vi "通用文件传.vi"(5 "原文件路径（使用对话框）":path) -> (2 "文本":string)   [LabVIEW 2016, in "数据传输系统-05.lvlib" / "自动更新.lvlib" / "TCP文件传输系统.lvlib" / "TCP发送文件.lvlib"]
panel:
  out "错误输出":errorcluster
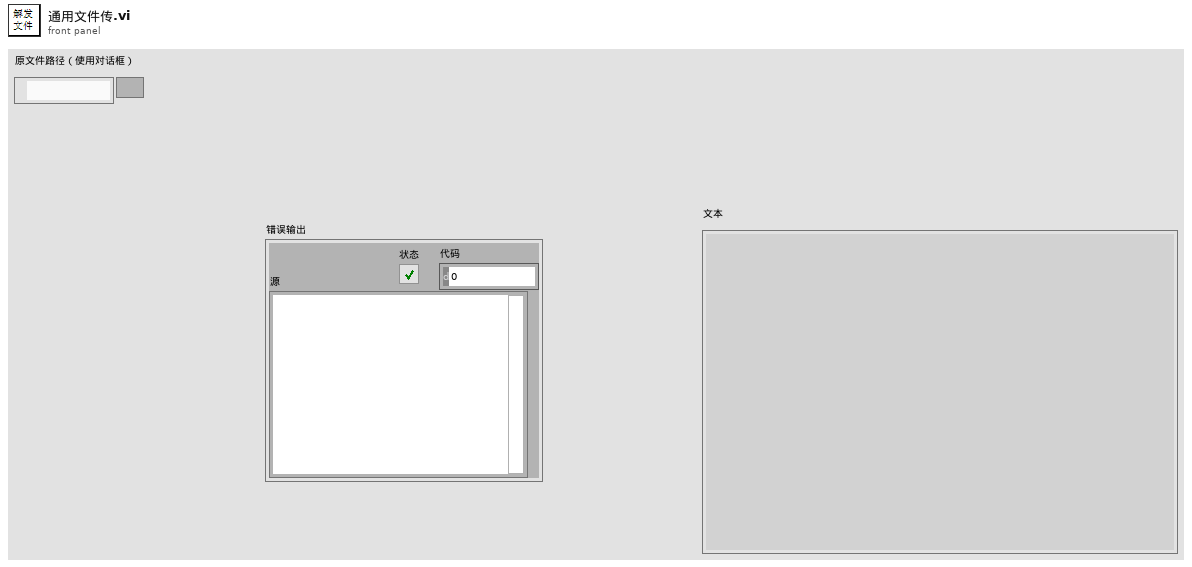
[diagram p1: front panel]
types:
  T1 = enum16{"big-endian, network order", "native, host order", "little-endian"}
  T2 = enum16{"open", "replace", "create", "open or create", "replace or create", "replace or create with confirmation"}
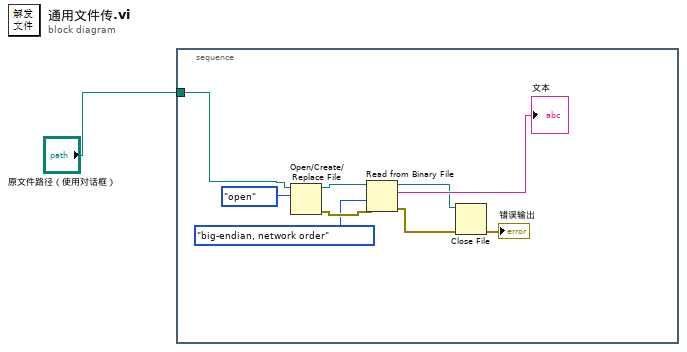
[diagram p0: block diagram]
diagram:
  n1 = stacked-sequence {
    tunnel: "原文件路径（使用对话框）" -> [w8]
    frame #0 {
      n2 = Open/Create/Replace File(file path (use dialog)=w8, operation (0:open)=T2."open" ("操作(0:open)")) -> (refnum out=w9:refnum<file>, error out=w6:errorcluster)  [unwired: 4 in, 1 out]
      n3 = Read from Binary File(8:w6, 9:T1."big-endian, network order" ("字节顺序(0:big-endian, network order)"), 11:w9) -> (0:w4:errorcluster, 2:→"文本":string, 3:w5:refnum<file>)  [unwired: 3 in, 1 out]
      n4 = Close File(refnum=w5, error in=w4) -> (error out=→"错误输出":errorcluster)  [unwired: 1 out]
    }
  }
